vi "Matrici lezione MC.vi"(1 "N":i16=4) -> (0 "2D Array":dbl[][](array[numeric]) format="%.2f")   [LabVIEW 2012]
doc: "M. Corti"
panel:
  out "Array":dbl[][][](array[numeric])
  in  "n° col.":i32=3
  out "vet riga 2":dbl[](array[numeric]) format="%.2f"
  out "Mat 2D":dbl[][](array[numeric]) format="%.2f"
  in  "n° righe":i32=2
  in  "n° quadri":i32=4
  out "element":dbl format="%.2f"
  out "Array  col":dbl[][](array[numeric]) format="%.2f"
  out "vet col":dbl[](array[numeric]) format="%.2f"
  out "vet riga-col":dbl[](array[numeric]) format="%.2f"
  out "vet riga":dbl[](array[numeric]) format="%.2f"
  out "Array  riga":dbl[][](array[numeric]) format="%.2f"
  out "1D array":dbl[](array[numeric]) format="%.2f"
  out "Array 3":dbl[](array[numeric]) format="%.2f"
  out "Array 2":dbl[](array[numeric]) format="%.2f"
  out "Array 1":dbl[](array[numeric]) format="%.2f"
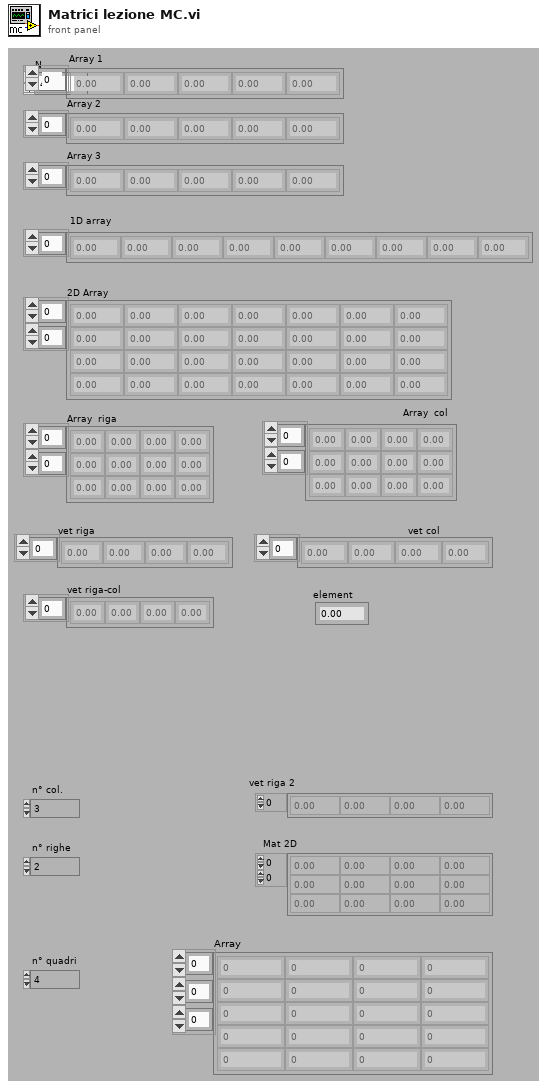
[diagram p1: front panel]
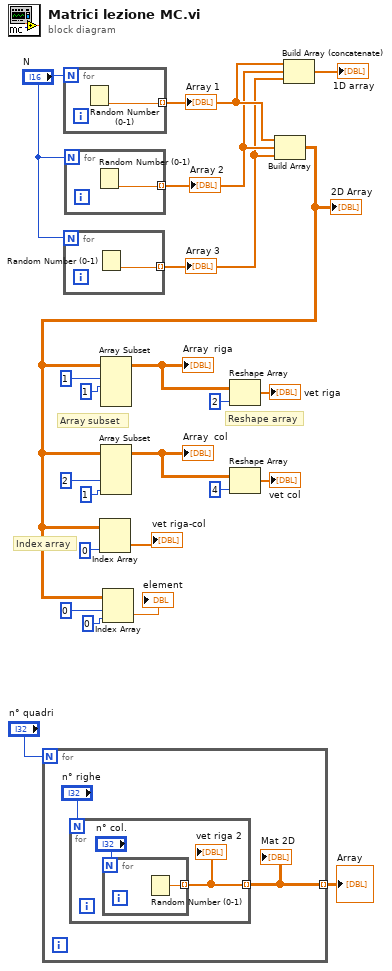
[diagram p0: block diagram]
diagram:
  # "Reshape array"
  # "Index array"
  # "Array subset"
  n1 = for {
    N: "n° quadri" -> [_]
    tunnel: [w24] -> w1 mode=indexing
    n2 = for {
      N: "n° righe" -> [_]
      tunnel: [w26] -> w24 mode=indexing
      n3 = for {
        N: "n° col." -> [_]
        tunnel: [w28] -> w26 mode=indexing
        n4 = Random Number (0-1)() -> (number: 0 to 1=w28:dbl)
      }
      "vet riga 2" <- w26
    }
    "Mat 2D" <- w24
  }
  "Array" <- w1
  n5 = for {
    N: "N" -> [_]
    tunnel: [w29] -> w6 mode=indexing
    n6 = Random Number (0-1)() -> (number: 0 to 1=w29:dbl)
  }
  "Array 1" <- w6
  n7 = for {
    N: "N" -> [_]
    tunnel: [w30] -> w4 mode=indexing
    n8 = Random Number (0-1)() -> (number: 0 to 1=w30:dbl)
  }
  "Array 3" <- w4
  n9 = for {
    N: "N" -> [_]
    tunnel: [w31] -> w5 mode=indexing
    n10 = Random Number (0-1)() -> (number: 0 to 1=w31:dbl)
  }
  "Array 2" <- w5
  n11 = Build Array(w6, w5, w4) -> (w10:dbl[][])
  "2D Array" <- w10
  n12 = Index Array(array=w10, index (col)=0 ("Disabled Index (col)")) -> (element=→"vet riga-col":dbl[])  [unwired: 1 in]
  n13 = Array Subset(array=w10, index (row)=1 ("Array Index"), length (row)=1 ("Array Length")) -> (w20:dbl[][])  [unwired: 2 in]
  "Array  riga" <- w20
  n14 = Array Subset(array=w10, index (col)=2 ("Array Index"), length (col)=1 ("Array Length")) -> (w15:dbl[][])  [unwired: 2 in]
  "Array  col" <- w15
  n15 = Index Array(array=w10, index (row)=0 ("Disabled Index (row)"), index (col)=0 ("Disabled Index (col)")) -> (element=→"element":dbl)
  n16 = Reshape Array(w20, 2 ("Dimension Size")) -> (→"vet riga":dbl[])
  n17 = Reshape Array(w15, 4 ("Dimension Size")) -> (→"vet col":dbl[])
  n18 = Build Array (concatenate)(w6, w5, w4) -> (→"1D array":dbl[])
